vi "State_Init_Data Map.vi"(8 "error in (no error)":errorcluster, 9 "Data":T1[](array[typedef]), 10 "Channel":string[](array[string]), 11 "shell in":refnum<class "launcher.lvclass">) -> (0 "error out":errorcluster, 1 "CVT Size":i32, 2 "Debug Message":string, 3 "shell out":refnum<class "launcher.lvclass">)   [LabVIEW 2021, in "launcher.lvclass"]
uses:
  launcher.lvclass
  C:/Program Files (x86)/National Instruments/LabVIEW 2021/user.lib/S2 Labs/Module Framework/Modules/Base/Module.lvclass
  <userlib>/S2 Labs/CVT Toolkit/TypeDefs/Data Cluster.ctl
  launcher.lvclass/launcher.ctl
  71d81f60-06b5-4f4e-b82e-b5bc43c3043b.vi
  Accessors/Read ch_alias.vi
  Accessors/Read ch_units.vi
  <userlib>/S2 Labs/CVT Toolkit/Variant Functions/Write Reserved Attributes.vi
  71d81f60-06b5-4f4e-b82e-b5bc43c3043b.vi/1291eb4c-788d-4886-9391-38aa82473be1.vi
  <userlib>/S2 Labs/CVT Toolkit/Variant Functions/Write Alias Attribute.vi
  <userlib>/S2 Labs/CVT Toolkit/Variant Functions/Write Unit Attribute.vi
  <userlib>/S2 Labs/CVT Toolkit/Variant Functions/Write Type Attribute.vi
  <userlib>/S2 Labs/CVT Toolkit/Variant Functions/Write Parms Attribute.vi
  <vilib>/JDP Science/JSONtext/Variant to JSON Text.vi
  <vilib>/JDP Science/JSONtext/LVClass Serializer/JSONtext LVClass Serializer.lvclass
  <userlib>/S2 Labs/Module Framework/Modules/Base/Module.lvclass
  <userlib>/S2 Labs/CVT Toolkit/CVT.lvclass
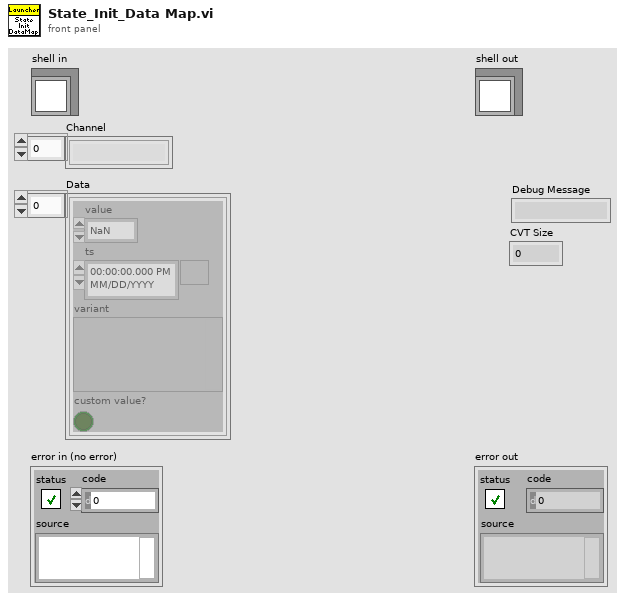
[diagram p1: front panel]
types:
  T1 = typedef "CVT.lvclass/Data Cluster.ctl" = cluster{"value":dbl, "ts":timestamp, "variant":variant, "custom value?":bool}
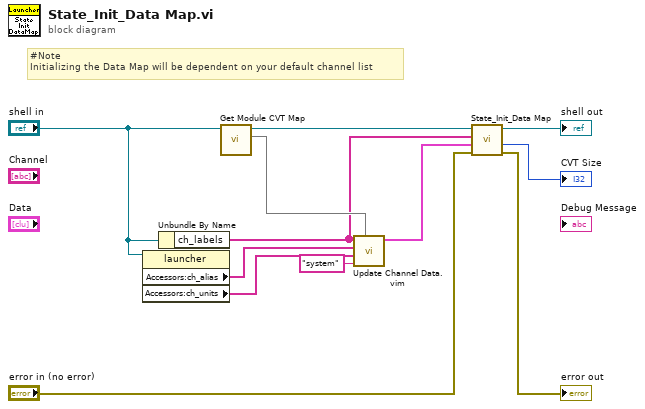
[diagram p0: block diagram]
diagram:
  # "#Note\nInitializing the Data Map will be dependent on your default channel list"
  n1 = property class="launcher"(reference="shell in") -> ("Accessors:ch_alias"=w2:string[], "Accessors:ch_units"=w1:string[])  [unwired: 1 in, 2 out]
  n2 = Unbundle By Name("shell in") -> ("ch_labels"=w5:string[])
  n3 = call <userlib>:"Get Module CVT Map.vi"("Module in"="shell in") -> ("CVT Data Map"=w8:map{string, T1}, "Module out"=w4:refnum<class "launcher.lvclass">)  [unwired: 8 in, 1 out]
  n4 = call "Update Channel Data.vim"("CVT Data Map"=w8, "type"="system", "unit"=w1, "alias"=w2, "ch labels"=w5) -> ("Data"=w6:T1[])  [unwired: 6 in]
  n5 = call-parent "State_Init_Data Map.vi"("error in (no error)"="error in (no error)", "Data"=w6, "Channel"=w5, "Module in"=w4) -> ("error out"=→"error out":errorcluster, "CVT Size"=→"CVT Size":i32, "Module out"=→"shell out":refnum<class "launcher.lvclass">)  [unwired: 4 in, 1 out]
